vi "Auton Script Builder.vi"(10 "Export?":bool) -> (3 "Export Successful?":bool)   [LabVIEW 2016]
uses:
  <vilib>/Utility/file.llb/Write Delimited Spreadsheet (DBL).vi
  <vilib>/Utility/file.llb/Read Delimited Spreadsheet (DBL).vi
  Robot Global Data.vi
panel:
  out "error out":errorcluster
  out "error out 2":errorcluster
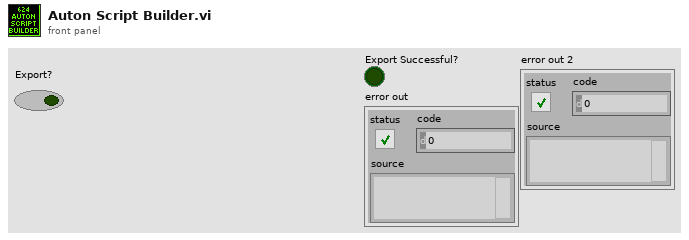
[diagram p1: front panel]
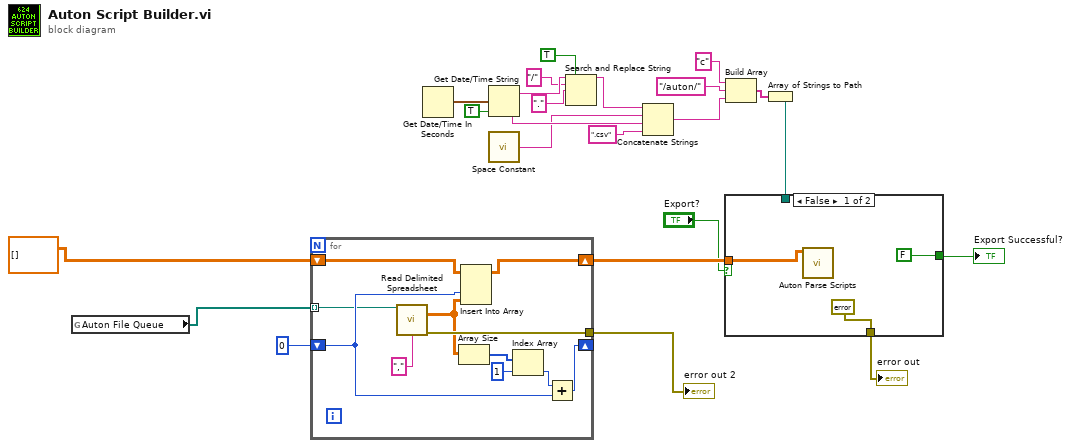
[diagram p0: block diagram]
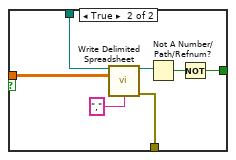
[diagram p2: hidden frame]
diagram:
  n1 = global read "Robot Global Data.vi" "Auton File Queue"() -> (w2:path[])
  n2 = for {
    shift-right: [w33] -> w22
    shift-left: dbl[][] [] -> [w34]
    tunnel: [w31] -> w11
    shift-right: [w26] -> _
    shift-left: 0 -> [w25]
    tunnel: w2 -> [w24] mode=indexing
    n3 = call-poly <vilib>:"Read Delimited Spreadsheet.vi"("file path (dialog if empty)"=w24, "delimiter (\\t)"="," ("delimiter (\\t)")) -> ("all rows"=w30:dbl[][], "error out"=w31:errorcluster)  [unwired: 8 in, 4 out]
    n4 = Array Size(array=w30) -> (size(s)=w29:i32[])
    n5 = Insert Into Array(array=w34, index (col)=w25, new element=w30) -> (w33:dbl[][])  [unwired: 1 in]
    n6 = Index Array(array=w29, index=1) -> (element=w27:i32)
    n7 = Add(x=w27, y=w25) -> (x+y=w26:i32)
  }
  "error out 2" <- w11
  n8 = Get Date/Time In Seconds() -> (seconds since 1Jan1904=w16:timestamp)
  n9 = Get Date/Time String(seconds (now)=w16, want seconds? (F)=TRUE) -> (date string=w8:string, time string=w14:string)  [unwired: 1 in]
  n10 = call <vilib>:"Space Constant.vi"() -> ("String"=w3:string)
  n11 = Search and Replace String(replace all?=TRUE ("replace all? (F)"), input string=w8, search string="/", replace string="." ("replace string (\"\")")) -> (result string=w4:string)  [unwired: 4 in, 3 out]
  n12 = Concatenate Strings(w4, w3, w14, ".csv" ("element")) -> (w12:string)
  n13 = Build Array("c", "/auton/", w12) -> (w18:string[])
  n14 = Array of Strings to Path(0:w18) -> (2:w17:path)  [unwired: 1 in]
  n15 = case shown="False" "Export?" {
    tunnel: w22 -> [w35 w44]
    tunnel: w17 -> [_ w43]
    tunnel: [FALSE w38] -> w1
    tunnel: [errorcluster {"status"=FALSE, "code"=0, "source"=""} ("error out") w39] -> w10
    frame False {
      n16 = call "Auton Parse Scripts.vi"("Array"=w35) -> ()  [unwired: 11 in]
    }
    frame True {
      n17 = call-poly <vilib>:"Write Delimited Spreadsheet.vi"("file path (dialog if empty)"=w43, "2D data"=w44, "delimiter (\\t)"="," ("delimiter (\\t)")) -> ("new file path (Not A Path if cancelled)"=w41:path, "error out"=w39:errorcluster)  [unwired: 11 in]
      n18 = Not A Number/Path/Refnum?(number/path/refnum=w41) -> (NaN/Path/Refnum?=w40:bool)
      n19 = Not(x=w40) -> (.not. x?=w38:bool)
    }
  }
  "Export Successful?" <- w1
  "error out" <- w10
